vi "GetDefaultParams.vi"(8 "error in (no error)":errorcluster, 11 "config file path":path) -> (0 "error out":errorcluster, 2 "DefaultINIParams":T1={"Handle"="", "eFunction"=0, "dRange"=0.0, "dResolution"=0.0, "eTriggerSource"=0, "dTriggerDelay"=0.0, "iMaxTimeMilliseconds"=0, "eMeasCompleteDest"=0, "iTriggerCount"=0, "iSampleCount"=0, "eSampleClock"=0, "dSampleInterval"=0.0, "iMaxTimeMillisecondsMultiPoint"=0, "iArraySize"=0, "dMinFreq"=0.0, "dMaxFreq"=0.0, "dFrequencyVoltageRange"=0.0, "eEdge"=10280, "sSource"="", "eEdgeSample"=10280, "sSourceSample"=""} {"eEdgeSample" items=["Rising"=10280, "Falling"=10171]; "eEdge" items=["Rising"=10280, "Falling"=10171]; "eSampleClock" items=["NULL"=0, "Immediate"=1, "External"=2, "Software Trigger"=3, "Interval"=10]; "eMeasCompleteDest" items=["None"=0, "External"=2]; "eTriggerSource" items=["NULL", "Immediate", "External", "Software Trigger"]; "eFunction" items=["NULL"=0, "DC Volts"=1, "AC Volts"=2, "DC Current"=3, "AC Current"=4, "Frequency"=104, "AC Coupled Direct Sampling"=1005]})   [LabVIEW 2014, in "SamplerPlugins.lvlib" / "SamplerPluginsBase.lvclass"]
uses:
  SamplerPluginsBase.lvclass
  TypeDefs/DefaultINIParams.ctl
  <vilib>/Utility/error.llb/Error Cluster From Error Code.vi
  <vilib>/ErrorRing/Error Ring.xnode
  <vilib>/Utility/config.llb/NI_LVConfig.lvlib
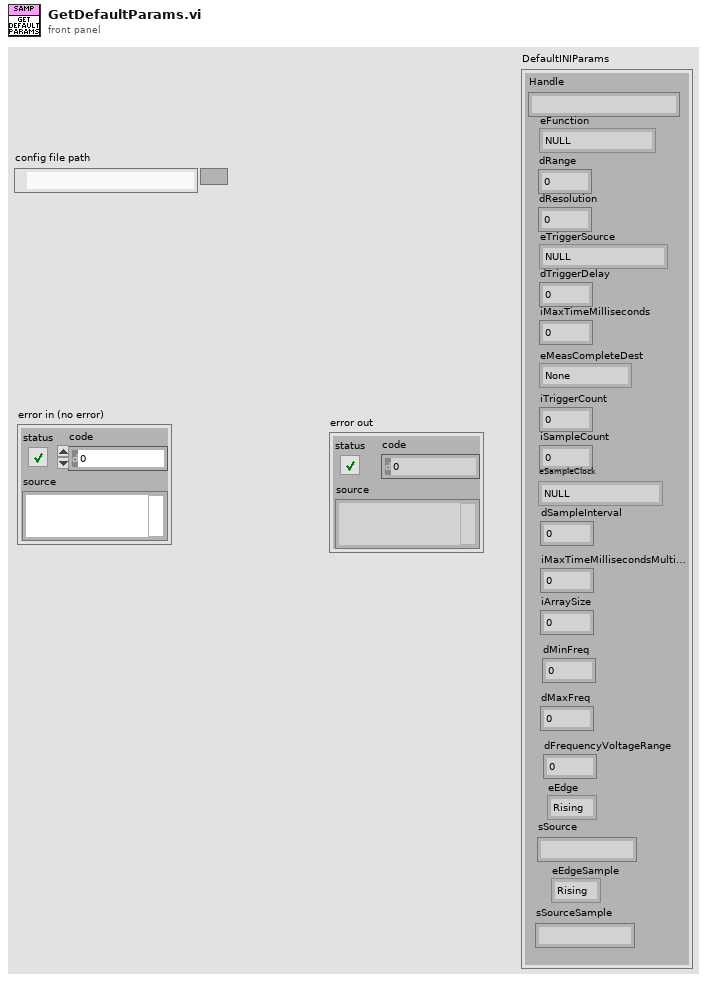
[diagram p1: front panel]
types:
  T1 = typedef "SamplerPlugins.lvlib/SamplerPluginsBase.lvclass/DefaultINIParams.ctl" = cluster{"Handle":string, "eFunction":u16, "dRange":dbl, "dResolution":dbl, "eTriggerSource":u16, "dTriggerDelay":dbl, "iMaxTimeMilliseconds":i32, "eMeasCompleteDest":u16, "iTriggerCount":i32, "iSampleCount":i32, "eSampleClock":u16, "dSampleInterval":dbl, "iMaxTimeMillisecondsMultiPoint":i32, "iArraySize":i32, "dMinFreq":dbl, "dMaxFreq":dbl, "dFrequencyVoltageRange":dbl, "eEdge":u16, "sSource":string, "eEdgeSample":u16, "sSourceSample":string}
  T2 = typedef "NI_LVConfig.lvlib/Config Data RefNum.ctl" = refnum<k1>
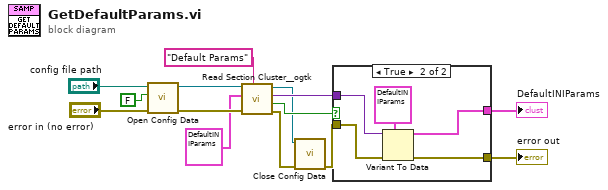
[diagram p0: block diagram]
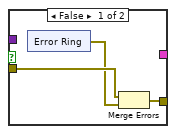
[diagram p2: hidden frame]
diagram:
  n1 = call <vilib>:"Open Config Data.vi"("error in (no error)"="error in (no error)", "create file if necessary (T)"=FALSE, "configuration file path"="config file path") -> ("error out"=w12:errorcluster, "refnum"=w11:T2)  [unwired: 6 in, 1 out]
  n2 = call <userlib>:"Read Section Cluster__ogtk.vi"("section (optional)"="Default Params", "error in (no error)"=w12, "Section Formatted Cluster Type"=T1 {"Handle"="", "eFunction"=0, "dRange"=0.0, "dResolution"=0.0, "eTriggerSource"=0, "dTriggerDelay"=0.0, "iMaxTimeMilliseconds"=0, "eMeasCompleteDest"=0, "iTriggerCount"=0, "iSampleCount"=0, "eSampleClock"=0, "dSampleInterval"=0.0, "iMaxTimeMillisecondsMultiPoint"=0, "iArraySize"=0, "dMinFreq"=0.0, "dMaxFreq"=0.0, "dFrequencyVoltageRange"=0.0, "eEdge"=10280, "sSource"="", "eEdgeSample"=10280, "sSourceSample"=""} ("DefaultINIParams"), "refnum"=w11) -> ("error out"=w4:errorcluster, "all found?"=w8:bool, "Section Formatted Cluster"=w7:variant, "dup refnum"=w2:T2)  [unwired: 3 in, 1 out]
  n3 = call <vilib>:"Close Config Data.vi"("error in (no error)"=w4, "refnum"=w2) -> ("error out"=w3:errorcluster)  [unwired: 8 in, 1 out]
  n4 = case shown="True" w8 {
    tunnel: w7 -> [_ w26]
    tunnel: w3 -> [w17 w25]
    tunnel: [_ w24] -> w6
    tunnel: [w15 w23] -> w1
    frame False {
      n5 = xnode "Error Ring"() -> ("error out"=w16:errorcluster)
      n6 = Merge Errors(w17, w16) -> (w15:errorcluster)
    }
    frame True {
      n7 = Variant To Data(error in=w25, type=T1 {"Handle"="", "eFunction"=0, "dRange"=0.0, "dResolution"=0.0, "eTriggerSource"=0, "dTriggerDelay"=0.0, "iMaxTimeMilliseconds"=0, "eMeasCompleteDest"=0, "iTriggerCount"=0, "iSampleCount"=0, "eSampleClock"=0, "dSampleInterval"=0.0, "iMaxTimeMillisecondsMultiPoint"=0, "iArraySize"=0, "dMinFreq"=0.0, "dMaxFreq"=0.0, "dFrequencyVoltageRange"=0.0, "eEdge"=10280, "sSource"="", "eEdgeSample"=10280, "sSourceSample"=""} ("DefaultINIParams"), Variant=w26) -> (data=w24:T1, error out=w23:errorcluster)
    }
  }
  "error out" <- w1
  "DefaultINIParams" <- w6
